vi "05.1-4 Config File on Event-driven SM.vi"() -> ()   [LabVIEW 2019]
uses:
  Support Files/03.2 States.ctl
  Support Files/05.1 Hardware Settings.ctl
  Support Files/03.2 State Machine Data.ctl
  Support Files/02.4 DAQmx Configuration Cluster.ctl
  <vilib>/DAQmx/write.llb/DAQmx Write (Analog DBL 1Chan 1Samp).vi
  <vilib>/Utility/file.llb/Write Delimited Spreadsheet (string).vi
  <vilib>/Utility/file.llb/Write Delimited Spreadsheet (DBL).vi
  <vilib>/DAQmx/create/channels.llb/DAQmx Create Channel (AO-Voltage-Basic).vi
  <vilib>/DAQmx/miscellaneous.llb/DAQmx Fill In Error Info.vi
panel:
  in  "Threshold (RMS)":dbl
  in  "Select Config File":bool
  in  "Generate Stimulus":bool
  in  "Acquire":bool
  out "Graph":dbl[][](graph)
  out "RMS Result per Channel":dbl[](array[numeric])
  out "Thershold Exceeded?":bool
  in  "Stop":bool
  in  "Clear":bool
  # "ANALYSIS"
  # "EVENTS"
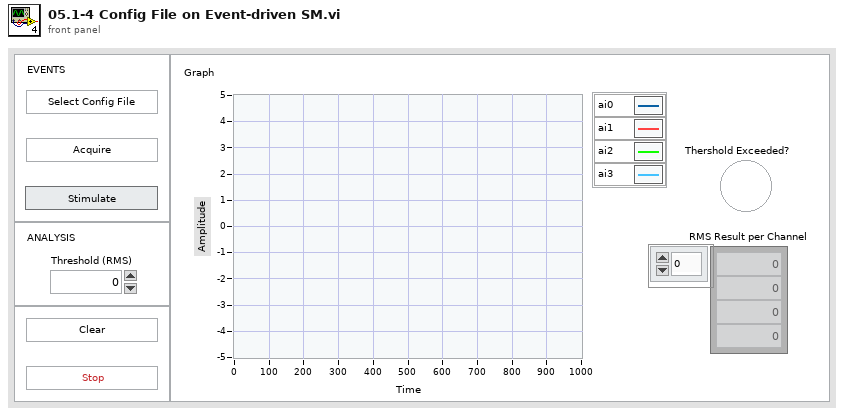
[diagram p1: front panel]
types:
  T1 = typedef "03.2 State Machine Data.ctl" = cluster{"Acquisition Data":dbl[][], "Stimulus?":bool}
  T2 = typedef "05.1 Hardware Settings.ctl" = cluster{"AI Channel":tag, "Sample Rate":dbl, "Samples per Channel":i32, "AO Channel":tag}
  T3 = typedef "03.2 States.ctl" = enum16{"Initialize", "Update UI", "Update Stimulus", "Wait for event", "Acquire", "Analyze", "Log", "Clear", "Shutdown"}
  T4 = typedef "02.4 DAQmx Configuration Cluster.ctl" = cluster{"Desired Sample Rate (Hz)":dbl, "sample mode":i32, "Minimum value":dbl, "Maximum value":dbl, "Physical Channel":tag, "units":i32, "thermocouple type":i32, "Samples per Channel":i32}
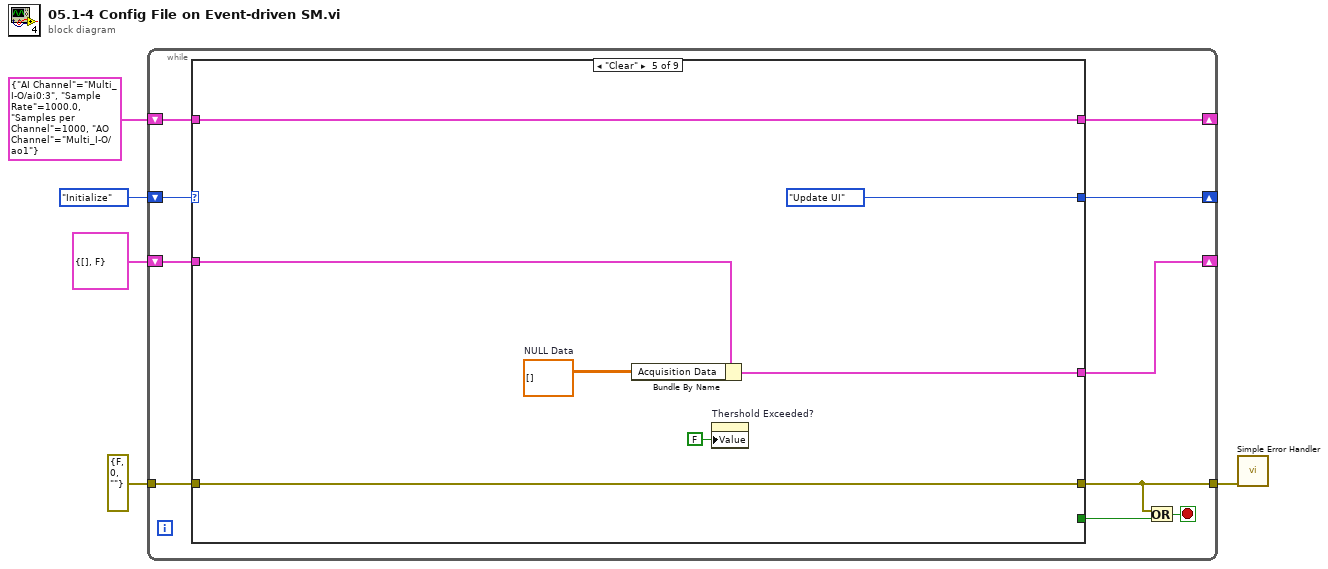
[diagram p0: block diagram]
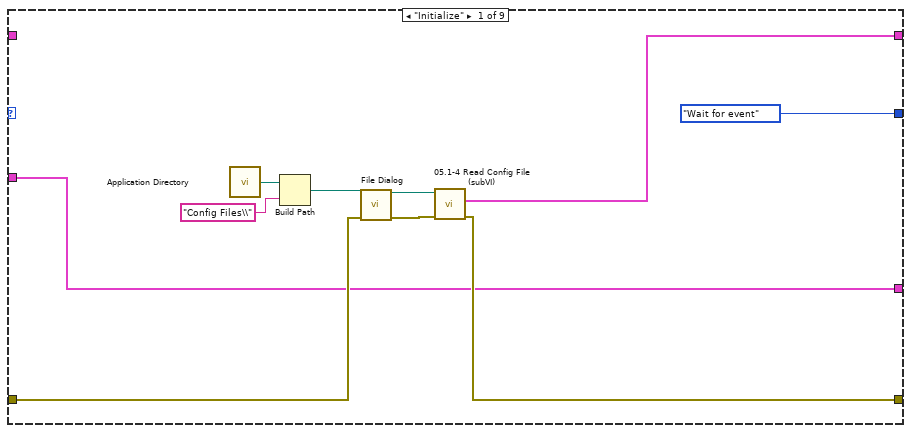
[diagram p2: hidden frame]
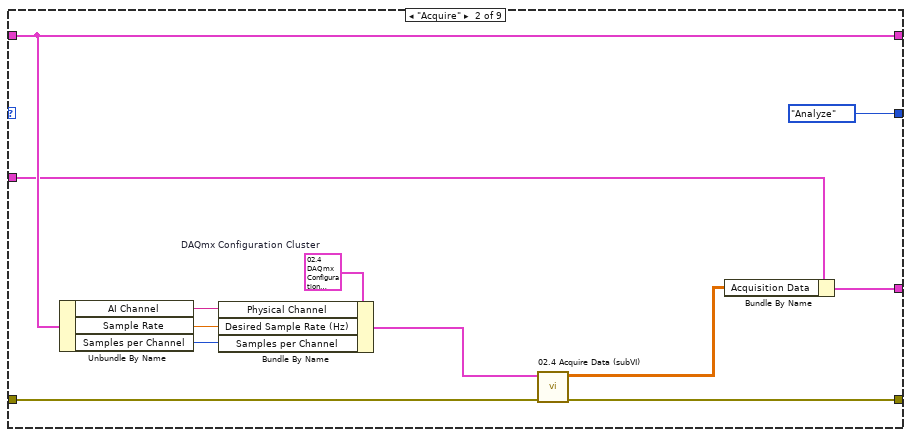
[diagram p3: hidden frame]
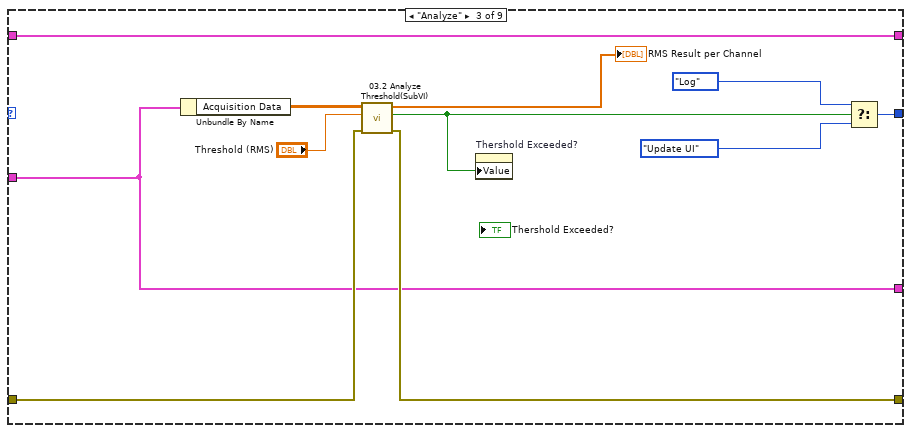
[diagram p4: hidden frame]
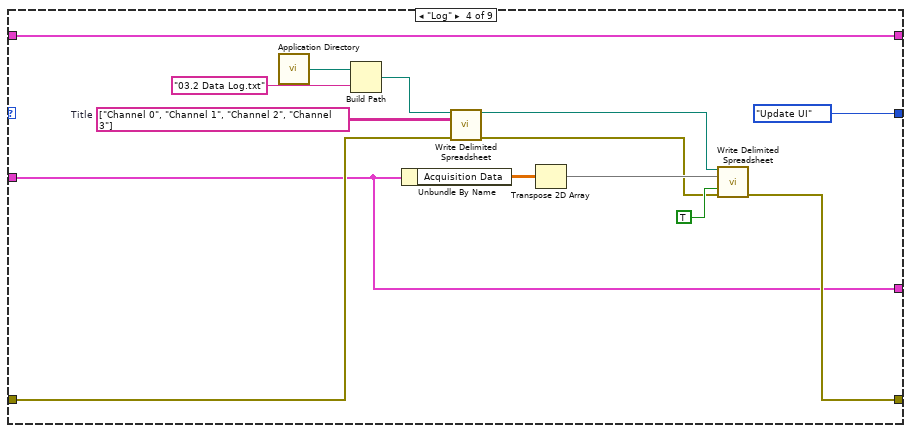
[diagram p5: hidden frame]
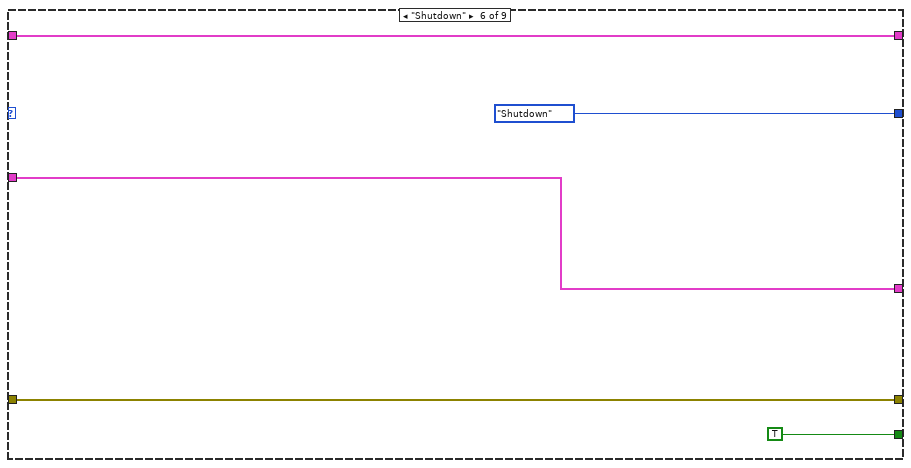
[diagram p6: hidden frame]
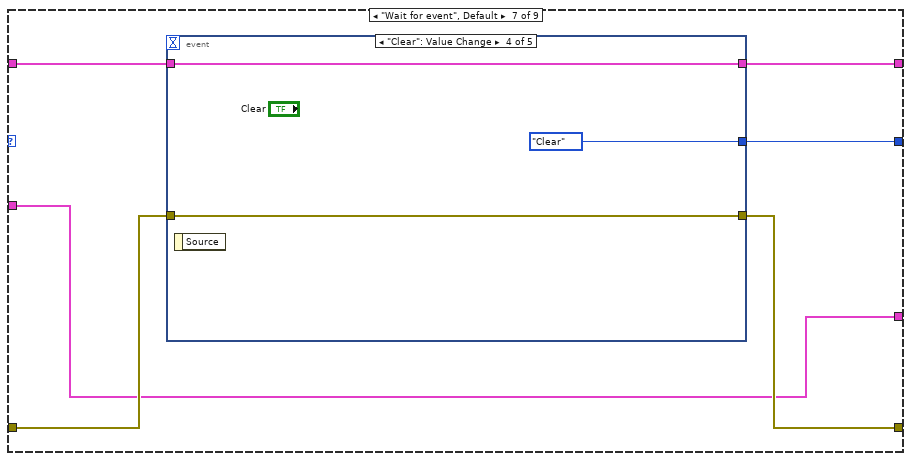
[diagram p7: hidden frame]
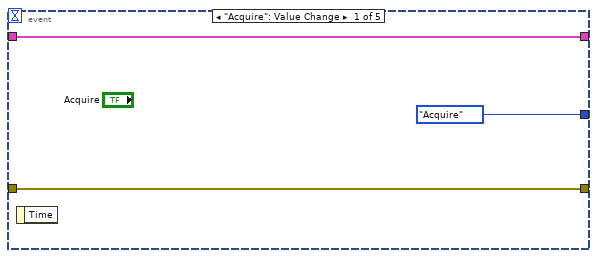
[diagram p8: hidden frame]
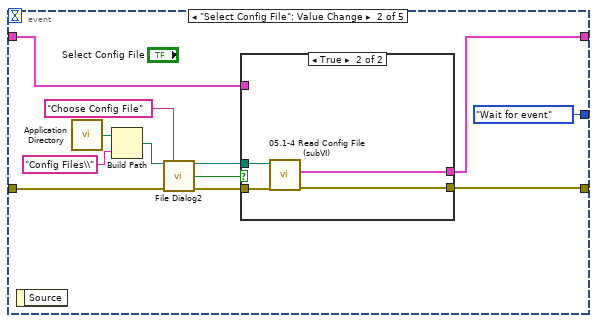
[diagram p9: hidden frame]
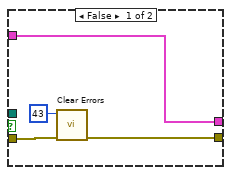
[diagram p10: hidden frame]
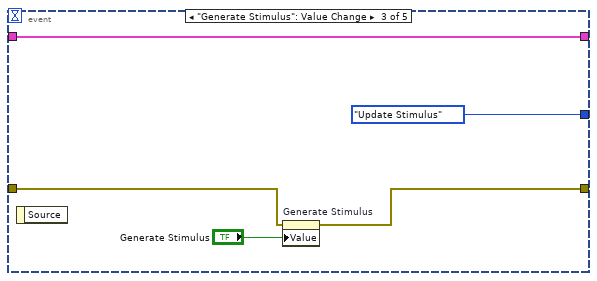
[diagram p11: hidden frame]
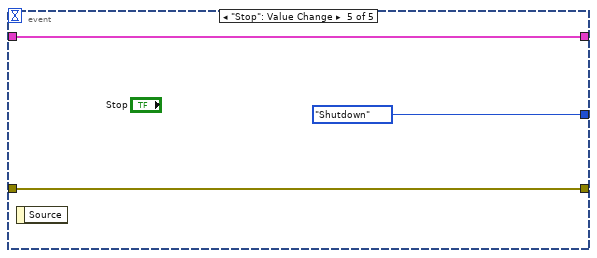
[diagram p12: hidden frame]
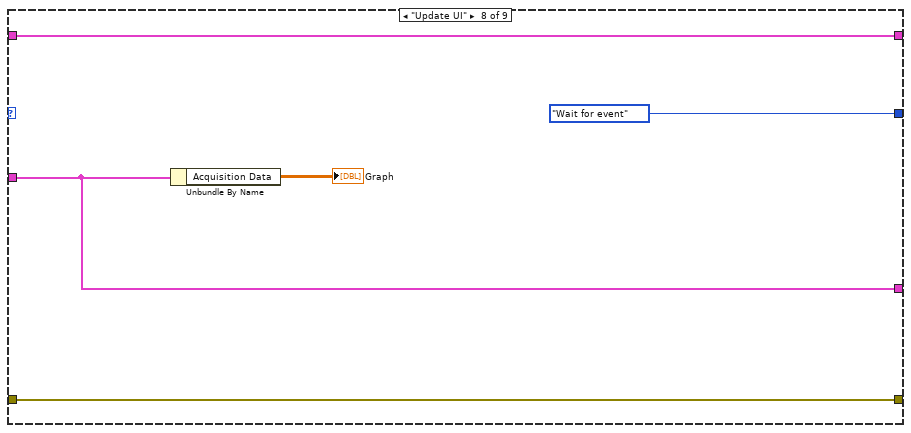
[diagram p13: hidden frame]
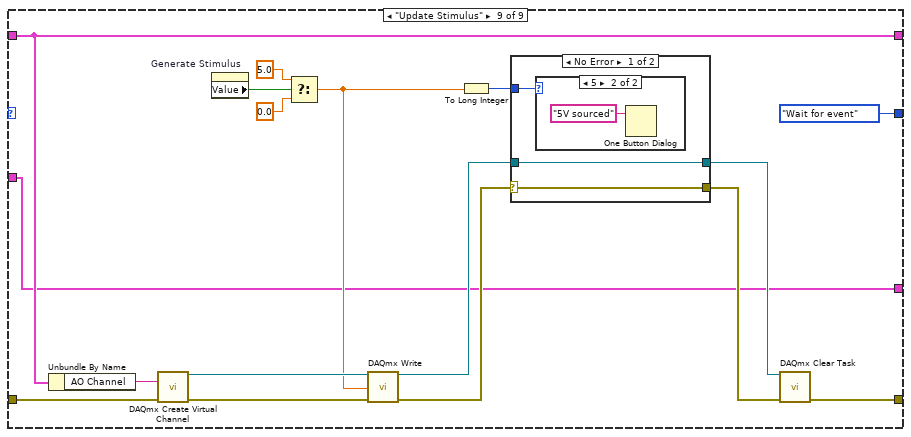
[diagram p14: hidden frame]
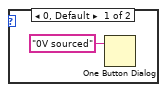
[diagram p15: hidden frame]
diagram:
  n1 = while {
    shift-right: [w14] -> _
    shift-left: 03.2_States."Initialize" ("State") -> [w15]
    tunnel: errorcluster {"status"=FALSE, "code"=0, "source"=""} ("error constant") -> [w13]
    tunnel: [w11] -> w3
    shift-right: [w8] -> _
    shift-left: T2 {"AI Channel"="Multi_I-O/ai0:3", "Sample Rate"=1000.0, "Samples per Channel"=1000, "AO Channel"="Multi_I-O/ao1"} ("Hardware Settings") -> [w10]
    shift-right: [w6] -> _
    shift-left: T1 {"Acquisition Data"=[], "Stimulus?"=FALSE} ("SM Data") -> [w7]
    stop <- w12 stop-if-true
    n2 = case shown="\"Clear\"" w15 {
      tunnel: [03.2_States."Wait for event" ("State") 03.2_States."Analyze" ("State") w47 03.2_States."Update UI" ("State") 03.2_States."Update UI" ("State") 03.2_States."Shutdown" ("State") w80 03.2_States."Wait for event" ("State") 03.2_States."Wait for event" ("State")] -> w14
      tunnel: [w18 w36 w43 w60 w68 w73 w79 w118 w126] -> w11
      tunnel: w13 -> [w21 w37 w44 w51 w68 w73 w78 w118 w136]
      tunnel: [w17 w29 w40 w49 w64 w70 w76 w116 w121] -> w8
      tunnel: w10 -> [_ w29 w40 w49 w64 w70 w77 w116 w121]
      tunnel: [_ _ _ _ _ TRUE _ _ _] -> w9
      tunnel: w7 -> [w16 w28 w39 w50 w67 w71 w75 w115 w120]
      tunnel: [w16 w26 w39 w50 w65 w71 w75 w115 w120] -> w6
      frame "Initialize" {
        n3 = call <vilib>:"Application Directory.vi"() -> ("Application Directory"=w24:path)
        n4 = Build Path(base path=w24, name or relative path="Config Files\\") -> (appended path=w22:path)
        n5 = call "File Dialog"("start path"=w22, "error in"=w21) -> ("selected path"=w19:path, "error out"=w20:errorcluster)  [unwired: 10 in, 2 out]
        n6 = call "05.1-4 Read Config File (subVI).vi"("Error In"=w20, "Config File In"=w19) -> ("Error Out"=w18:errorcluster, "Hardware Settings"=w17:T2)  [unwired: 7 in, 1 out]
      }
      frame "Acquire" {
        w34 = T4 {"Desired Sample Rate (Hz)"=-1.0, "sample mode"=10178, "Minimum value"=-1.0, "Maximum value"=-1.0, "Physical Channel"="", "units"=10143, "thermocouple type"=10072, "Samples per Channel"=0}  # DAQmx Configuration Cluster
        n7 = Unbundle By Name(w29) -> ("AI Channel"=w33:tag, "Sample Rate"=w32:dbl, "Samples per Channel"=w31:i32)
        n8 = Bundle By Name(cluster=w34, "Physical Channel"=w33, "Desired Sample Rate (Hz)"=w32, "Samples per Channel"=w31) -> (w30:T4)
        n9 = call "02.4 Acquire Data (subVI).vi"("Error In"=w37, "DAQmx Configuration Cluster"=w30) -> ("error out"=w36:errorcluster, "2D DBL"=w27:dbl[][])  [unwired: 8 in]
        n10 = Bundle By Name(cluster=w28, "Acquisition Data"=w27) -> (w26:T1)
      }
      frame "Analyze" {
        n11 = Unbundle By Name(w39) -> ("Acquisition Data"=w48:dbl[][])
        n12 = call "03.2 Analyze Threshold(SubVI).vi"("Error In"=w44, "Threshold (RMS)"="Threshold (RMS)", "Data"=w48) -> ("Error Out"=w43:errorcluster, "Threshold exceeded?"=w38:bool, "RMS Results per Channel"=→"RMS Result per Channel":dbl[])  [unwired: 6 in]
        n13 = property on="Thershold Exceeded?" class="Bool (strict)"("Value"=w38) -> ()  [unwired: 2 in, 2 out]
        n14 = Select(t=03.2_States."Log" ("State"), s=w38, f=03.2_States."Update UI" ("State")) -> (s? t:f=w47:T3)
      }
      frame "Log" {
        w53 = string[][] [["Channel 0", "Channel 1", "Channel 2", "Channel 3"]]  # Title
        n15 = call <vilib>:"Application Directory.vi"() -> ("Application Directory"=w62:path)
        n16 = Build Path(base path=w62, name or relative path="03.2 Data Log.txt") -> (appended path=w54:path)
        n17 = Unbundle By Name(w50) -> ("Acquisition Data"=w58:dbl[][])
        n18 = call-poly <vilib>:"Write Delimited Spreadsheet.vi"("file path (dialog if empty)"=w54, "2D data"=w53, "error in (no error)"=w51) -> ("new file path (Not A Path if cancelled)"=w56:path, "error out"=w52:errorcluster)  [unwired: 11 in]
        n19 = Transpose 2D Array(2D array=w58) -> (transposed array=w57:dbl[][])
        n20 = call-poly <vilib>:"Write Delimited Spreadsheet.vi"("file path (dialog if empty)"=w56, "2D data"=w57, "append to file? (new file:F)"=TRUE, "error in (no error)"=w52) -> ("error out"=w60:errorcluster)  [unwired: 10 in, 1 out]
      }
      frame "Clear" {
        w66 = dbl[][] []  # NULL Data
        n21 = Bundle By Name(cluster=w67, "Acquisition Data"=w66) -> (w65:T1)
        n22 = property on="Thershold Exceeded?" class="Bool (strict)"("Value"=FALSE ("Thershold Exceeded?")) -> ()  [unwired: 2 in, 2 out]
      }
      frame "Shutdown" {
      }
      frame "Wait for event", Default {
        n23 = event shown="[3] \"Clear\": Value Change" {
          selector: _ -> [_ _ _ _ _]
          dyn-events: _ -> [_ _ _ _ _]
          timeout: _ -> [_ _ _ _ _]
          tunnel: [03.2_States."Acquire" ("State") 03.2_States."Wait for event" ("State") 03.2_States."Update Stimulus" ("State") 03.2_States."Clear" ("State") 03.2_States."Shutdown" ("State")] -> w80
          tunnel: [w82 w88 w104 w109 w112] -> w79
          tunnel: w78 -> [w82 w92 w105 w109 w112]
          tunnel: [w81 w87 w107 w111 w113] -> w76
          tunnel: w77 -> [w81 w85 w107 w111 w113]
          event "Acquire": Value Change {
            n24 = event-data() -> ()  [unwired: 1 in, 1 out]
          }
          event "Select Config File": Value Change {
            n25 = event-data() -> ()  [unwired: 1 in, 1 out]
            n26 = call <vilib>:"Application Directory.vi"() -> ("Application Directory"=w91:path)
            n27 = Build Path(base path=w91, name or relative path="Config Files\\") -> (appended path=w89:path)
            n28 = call "File Dialog2"("start path"=w89, "prompt"="Choose Config File", "error in"=w92) -> ("selected path"=w94:path, "exists"=w95:bool, "error out"=w93:errorcluster)  [unwired: 9 in, 1 out]
            n29 = case shown="True" w95 {
              tunnel: w94 -> [_ w103]
              tunnel: w93 -> [w98 w102]
              tunnel: [w97 w101] -> w88
              tunnel: [w96 w100] -> w87
              tunnel: w85 -> [w96 _]
              frame False {
                n30 = call <vilib>:"Clear Errors.vi"("error in (no error)"=w98, "specific error code to clear (0: all)"=43) -> ("error out"=w97:errorcluster)  [unwired: 4 in, 1 out]
              }
              frame True {
                n31 = call "05.1-4 Read Config File (subVI).vi"("Error In"=w102, "Config File In"=w103) -> ("Error Out"=w101:errorcluster, "Hardware Settings"=w100:T2)  [unwired: 7 in, 1 out]
              }
            }
          }
          event "Generate Stimulus": Value Change {
            n32 = event-data() -> ()  [unwired: 1 in, 1 out]
            n33 = property on="Generate Stimulus" class="Bool (strict)"(error in=w105, "Value"="Generate Stimulus") -> (error out=w104:errorcluster)  [unwired: 1 in, 1 out]
          }
          event "Clear": Value Change {
            n34 = event-data() -> ()  [unwired: 1 in, 1 out]
          }
          event "Stop": Value Change {
            n35 = event-data() -> ()  [unwired: 1 in, 1 out]
          }
        }
      }
      frame "Update UI" {
        n36 = Unbundle By Name(w115) -> ("Acquisition Data"=→"Graph":dbl[][])
      }
      frame "Update Stimulus" {
        n37 = Unbundle By Name(w121) -> ("AO Channel"=w122:tag)
        n38 = call-poly <vilib>:"DAQmx Create Virtual Channel.vi"("physical channels"=w122, "error in"=w136) -> ("task out"=w134:refnum<k21>, "error out"=w135:errorcluster)  [unwired: 12 in]
        n39 = property on="Generate Stimulus" class="Bool (strict)"() -> ("Value"=w123:bool)  [unwired: 2 in, 2 out]
        n40 = Select(t=5.0, s=w123, f=0.0) -> (s? t:f=w131:dbl)
        n41 = call-poly <vilib>:"DAQmx Write.vi"("task/channels in"=w134, "data"=w131, "error in"=w135) -> ("task out"=w129:refnum<k21>, "error out"=w130:errorcluster)  [unwired: 10 in, 1 out]
        n42 = To Long Integer(number=w131) -> (32bit integer=w124:i32)
        n43 = case shown="No Error" w130 {
          selector: w130 -> [w139 w142]
          tunnel: w129 -> [w138 w143]
          tunnel: [w139 w142] -> w128
          tunnel: [w138 w143] -> w127
          tunnel: w124 -> [w137 _]
          frame No Error {
            n44 = case shown="5" w137 {
              frame 0, Default {
                n45 = One Button Dialog(message="0V sourced") -> ()  [unwired: 1 in, 1 out]
              }
              frame 5 {
                n46 = One Button Dialog(message="5V sourced") -> ()  [unwired: 1 in, 1 out]
              }
            }
          }
          frame Error {
          }
        }
        n47 = call <vilib>:"DAQmx Clear Task.vi"("task in"=w127, "error in"=w128) -> ("error out"=w126:errorcluster)  [unwired: 13 in]
      }
    }
    n48 = Or(x=w11, y=w9) -> (x .or. y?=w12:bool)
  }
  n49 = call <vilib>:"Simple Error Handler.vi"("error in (no error)"=w3) -> ()  [unwired: 4 in, 5 out]
